vi "Close.vi"(8 "error in (no error)":errorcluster, 11 "Module Data In":refnum<class "Rename.lvclass">) -> (0 "error out":errorcluster, 3 "Module Data Out":refnum<class "Rename.lvclass">)   [LabVIEW 2015, in "Generic Module Library.lvlib" / "Template G_Module.lvlib" / "Rename.lvclass"]
uses:
  Rename.lvclass
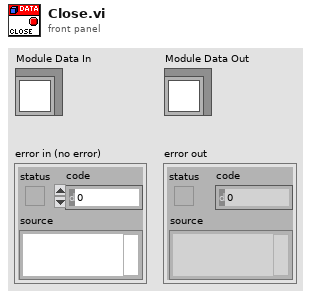
[diagram p1: front panel]
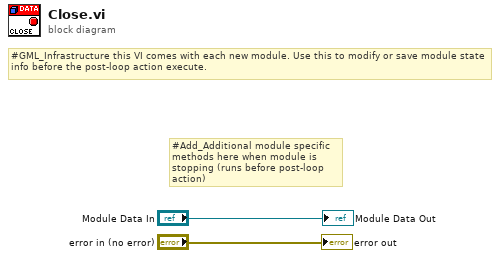
[diagram p0: block diagram]
diagram:
  # "#GML_Infrastructure this VI comes with each new module. Use this to modify or save module state info before the post-loop action execute."
  # "#Add_Additional module specific methods here when module is stopping (runs before post-loop action)"
  "error out" <- "error in (no error)"
  "Module Data Out" <- "Module Data In"
